vi "tipclean.vi"(8 "error in (no error)":errorcluster, 11 "Input":string="34,45,89") -> (0 "error out":errorcluster, 3 "Output":string)   [LabVIEW 2014]
uses:
  <userlib>/Nanonis Prog Interface V5/Nanonis Prog Interface.lvlib
panel:
  out "crashed?":bool
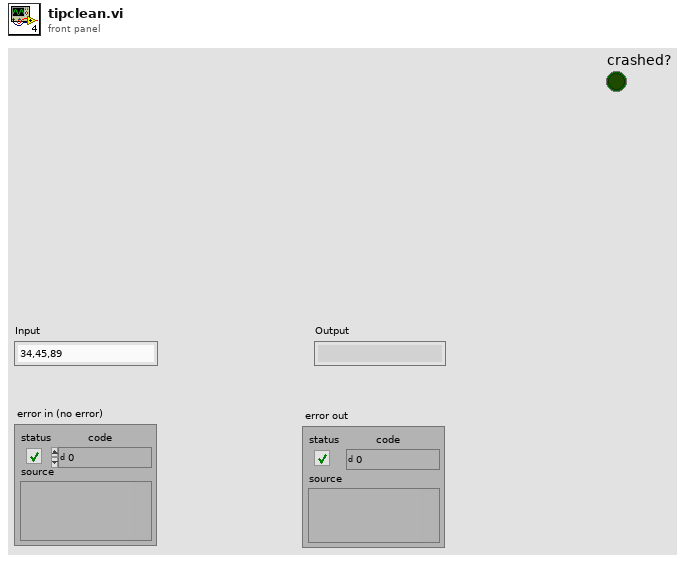
[diagram p1: front panel]
types:
  T1 = enum8{"Group 1", "Group 2", "Group 3", "Group 4", "Group 5", "Group 6"}
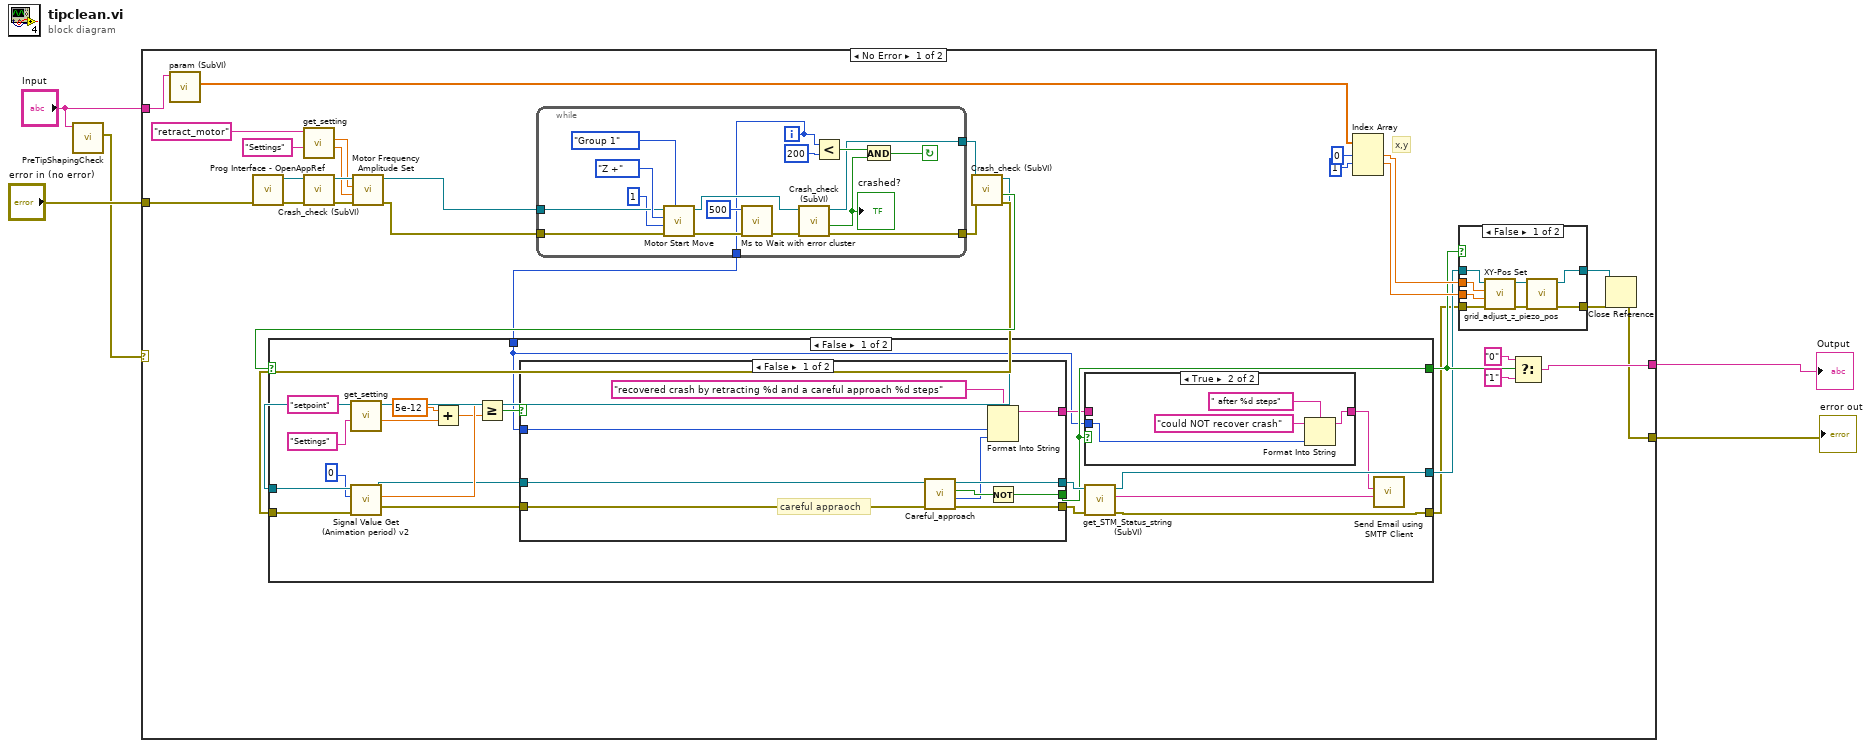
[diagram p0: block diagram]
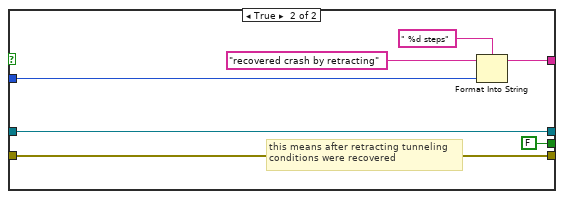
[diagram p4: hidden frame]
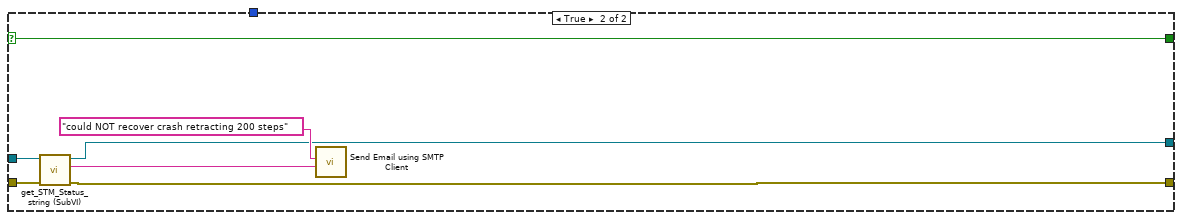
[diagram p5: hidden frame]
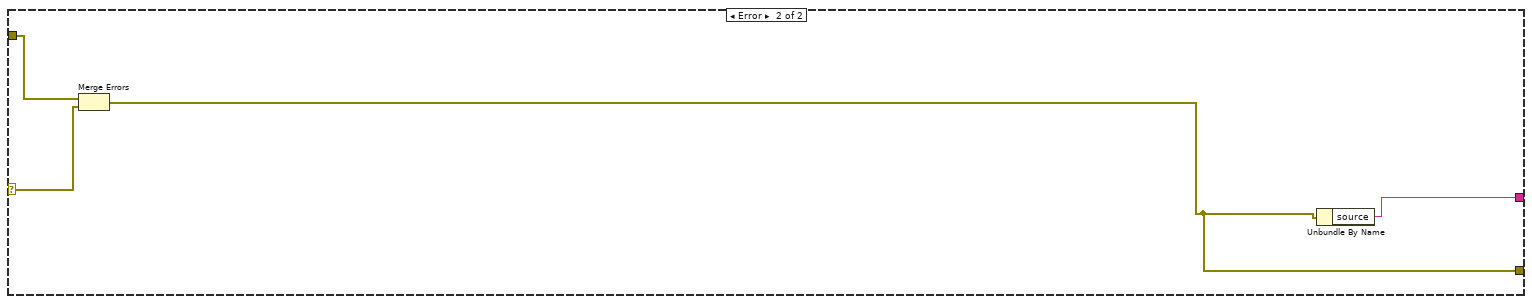
[diagram p6: hidden frame]
diagram:
  n1 = call "PreTipShapingCheck.vi"("Input"="Input") -> ("Error"=w2:errorcluster)  [unwired: 8 in, 2 out]
  n2 = case shown="No Error" w2 {
    selector: w2 -> [_ w116]
    tunnel: [w37 w114] -> w5
    tunnel: "error in (no error)" -> [w36 w117]
    tunnel: [w35 w115] -> w3
    tunnel: "Input" -> [w13 _]
    frame No Error {
      # "x,y"
      n3 = call <userlib>:"param (SubVI).vi"("Input"=w13) -> ("parm"=w16:dbl[])  [unwired: 8 in, 2 out]
      n4 = call <userlib>:"Prog Interface - OpenAppRef.vi"("Error in (no error)"=w36) -> ("Error out"=w33:errorcluster, "Application reference"=w34:refnum<vi>)  [unwired: 5 in]
      n5 = call "get_setting.vi"("section"="Settings", "key"="retract_motor") -> ("output 2"=w25:dbl, "output 1"=w26:dbl)  [unwired: 5 in, 3 out]
      n6 = call "Crash_check (SubVI).vi"("error in (no error)"=w33, "Application in"=w34) -> ("error out"=w28:errorcluster, "Application out"=w27:refnum<vi>)  [unwired: 7 in, 1 out]
      n7 = call <userlib>:"Motor Frequency Amplitude Set.vi"("Error in (no error)"=w28, "Amplitude (V) (NaN=no change)"=w25, "Frequency (Hz) (NaN=no change)"=w26, "Application ref in"=w27) -> ("Error out"=w23:errorcluster, "Application ref out"=w24:refnum<vi>)  [unwired: 6 in]
      n8 = while {
        tunnel: w24 -> [w111]
        tunnel: w23 -> [w110]
        tunnel: [w100] -> w22
        tunnel: [w99] -> w21
        tunnel: [w98] -> w17
        i -> [w98]
        stop <- w102 continue-if-true
        n9 = call <userlib>:"Motor Start Move.vi"("Group"=T1."Group 1", "Error in (no error)"=w110, "Number of steps"=u16 1, "Direction"=enum16{"X +", "X -", "Y +", "Y -", "Z +", "Z -"}."Z +", "Application ref in"=w111) -> ("Error out"=w106:errorcluster, "Application ref out"=w108:refnum<vi>)  [unwired: 4 in]
        n10 = call <userlib>:"Ms to Wait with error cluster.vi"("error in (no error)"=w106, "milliseconds to wait"=u32 500) -> ("error out"=w105:errorcluster)  [unwired: 4 in, 1 out]
        n11 = call "Crash_check (SubVI).vi"("error in (no error)"=w105, "Application in"=w108) -> ("error out"=w100:errorcluster, "crashed?"=w107:bool, "Application out"=w99:refnum<vi>)  [unwired: 7 in]
        "crashed?" <- w107
        n12 = Less?(x=w98, y=200) -> (x < y?=w101:bool)
        n13 = And(x=w101, y=w107) -> (x .and. y?=w102:bool)
      }
      n14 = call "Crash_check (SubVI).vi"("error in (no error)"=w22, "Application in"=w21) -> ("error out"=w19:errorcluster, "crashed?"=w20:bool, "Application out"=w18:refnum<vi>)  [unwired: 7 in]
      n15 = case shown="False" w20 {
        selector: w20 -> [_ w97]
        tunnel: w19 -> [w66 w93]
        tunnel: w18 -> [w65 w95]
        tunnel: [w50 w97] -> w10
        tunnel: [w55 w94] -> w9
        tunnel: [w53 w92] -> w8
        tunnel: w17 -> [w48 _]
        frame False {
          n16 = call "get_setting.vi"("section"="Settings", "key"="setpoint") -> ("output 2"=w62:dbl)  [unwired: 5 in, 4 out]
          n17 = call <userlib>:"Signal Value Get (Animation period) v2.vi"("error in (no error)"=w66, "Signal index (0-79)"=i8 0, "Application ref in"=w65) -> ("error out"=w57:errorcluster, "Signal value"=w63:sgl, "Application ref out"=w58:refnum<vi>)  [unwired: 5 in]
          n18 = Add(x=5e-12, y=w62) -> (x+y=w61:dbl)
          n19 = Greater Or Equal?(x=w63, y=w61) -> (x >= y?=w59:bool)
          n20 = case shown="False" w59 {
            tunnel: [w78 FALSE] -> w50
            tunnel: w58 -> [w83 w88]
            tunnel: w57 -> [w82 w89]
            tunnel: [w81 w88] -> w56
            tunnel: [w80 w89] -> w54
            tunnel: [w77 w86] -> w49
            tunnel: w48 -> [w75 w85]
            frame False {
              # "careful appraoch"
              n21 = call "Careful_approach.vi"("Error in (no error)"=w82, "Application ref in"=w83) -> ("Error out"=w80:errorcluster, "steps_taken"=w74:i32, "approached?"=w79:bool, "Application ref out"=w81:refnum<vi>)  [unwired: 6 in]
              n22 = Format Into String(format string="recovered crash by retracting %d and a careful approach %d steps" ("Subject"), w75, w74) -> (resulting string=w77:string)  [unwired: 2 in, 1 out]
              n23 = Not(x=w79) -> (.not. x?=w78:bool)
            }
            frame True {
              # "this means after retracting tunneling\nconditions were recovered"
              n24 = Format Into String(format string=" %d steps", initial string="recovered crash by retracting" ("Subject"), w85) -> (resulting string=w86:string)  [unwired: 1 in, 1 out]
            }
          }
          n25 = case shown="True" w50 {
            tunnel: [w69 w72] -> w51
            tunnel: w49 -> [w69 _]
            tunnel: w48 -> [_ w71]
            frame False {
            }
            frame True {
              n26 = Format Into String(format string=" after %d steps", initial string="could NOT recover crash" ("Subject"), w71) -> (resulting string=w72:string)  [unwired: 1 in, 1 out]
            }
          }
          n27 = call "get_STM_Status_string (SubVI).vi"("error in (no error)"=w54, "Application in"=w56) -> ("error out"=w53:errorcluster, "JSON string"=w52:string, "Application out"=w55:refnum<vi>)  [unwired: 7 in]
          n28 = call "Send Email using SMTP Client.vi"("Message"=w52, "subject"=w51) -> ()  [unwired: 9 in, 1 out]
        }
        frame True {
          n29 = call "get_STM_Status_string (SubVI).vi"("error in (no error)"=w93, "Application in"=w95) -> ("error out"=w92:errorcluster, "JSON string"=w91:string, "Application out"=w94:refnum<vi>)  [unwired: 7 in]
          n30 = call "Send Email using SMTP Client.vi"("Message"=w91, "subject"="could NOT recover crash retracting 200 steps" ("Subject")) -> ()  [unwired: 9 in, 1 out]
        }
      }
      n31 = Index Array(array=w16, index #1=0 ("index"), index #2=1 ("index")) -> (element #1=w12:dbl, element #2=w11:dbl)  [unwired: 1 in, 1 out]
      n32 = case shown="False" w10 {
        tunnel: w12 -> [w45 _]
        tunnel: w11 -> [w44 _]
        tunnel: w9 -> [w43 w47]
        tunnel: w8 -> [w42 w46]
        tunnel: [w38 w46] -> w7
        tunnel: [w41 w47] -> w6
        frame False {
          n33 = call <userlib>:"XY-Pos Set.vi"("error in (no error)"=w42, "Y (m)"=w44, "X (m)"=w45, "Application ref in"=w43) -> ("error out"=w39:errorcluster, "Application ref out"=w40:refnum<vi>)  [unwired: 4 in]
          n34 = call "grid_adjust_z_piezo_pos.vi"("Error in (no error)"=w39, "Application ref in"=w40) -> ("Error out"=w38:errorcluster, "Application ref out"=w41:refnum<vi>)  [unwired: 8 in]
        }
        frame True {
        }
      }
      n35 = Select(t="0", s=w10, f="1") -> (s? t:f=w37:string)
      n36 = Close Reference(reference=w6, error in (no error)=w7) -> (error out=w35:errorcluster)
    }
    frame Error {
      n37 = Merge Errors(w117, w116) -> (w115:errorcluster)
      n38 = Unbundle By Name(w115) -> ("source"=w114:string)
    }
  }
  "Output" <- w5
  "error out" <- w3
